vi "TCP_SetControl.vi"(0 "VI Refnum":refnum<vi>, 1 "Input":string, 3 "error in (no error)":errorcluster) -> (8 "Found?":bool, 10 "error out":errorcluster)   [LabVIEW 2019]
uses:
  <vilib>/Utility/Data Type/NI_Data Type.lvlib
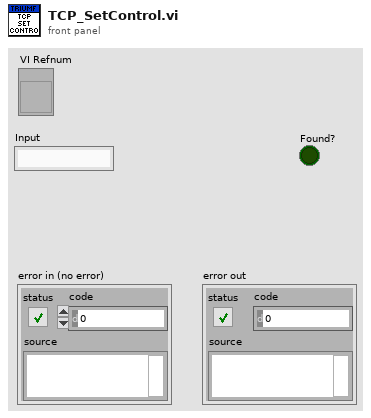
[diagram p1: front panel]
types:
  T1 = typedef "NI_Data Type.lvlib/Data Type.ctl" = enum8{"Invalid Type", "Void", "I8", "I16", "I32", "I64", "U8", "U16", "U32", "U64", "Single Float", "Double Float", "Extended Float", "Single Complex", "Double Complex", "Extended Complex", "Enum U8", "Enum U16", "Enum U32", "Enum U64", "Single Float With Unit", "Double Float With Unit", "Extended Float With Unit", "Single Complex with Unit", "Double Complex with Unit", "Extended Complex with Unit", "Boolean", "String", "Path", "Picture", "Tag", "Array", "Cluster", "Variant", "LV Variant", "Waveform", "Timestamp", "Digital Waveform", "Digital Data", "ExpressData", "Refnum", "External Data", "VI", "Poly VI", "LabVIEW Class Instance", "Fixed Point", "Set Collection", "Map Collection"}
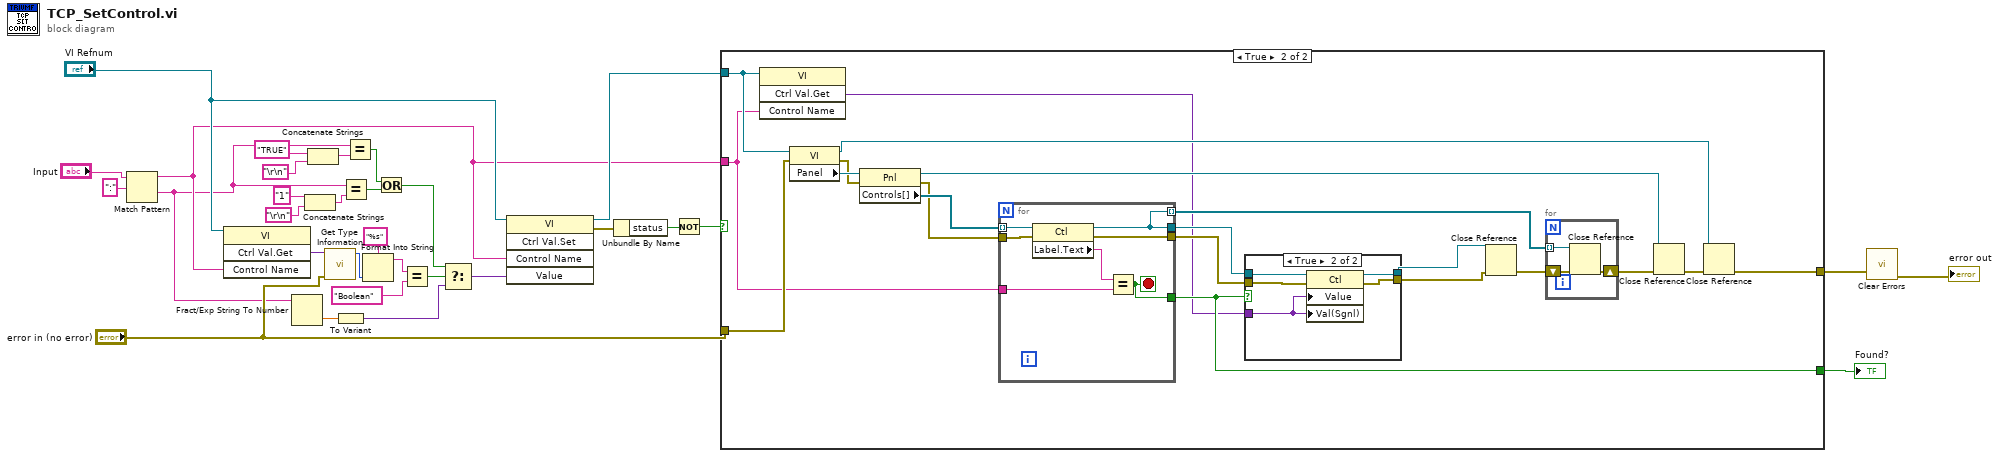
[diagram p0: block diagram]
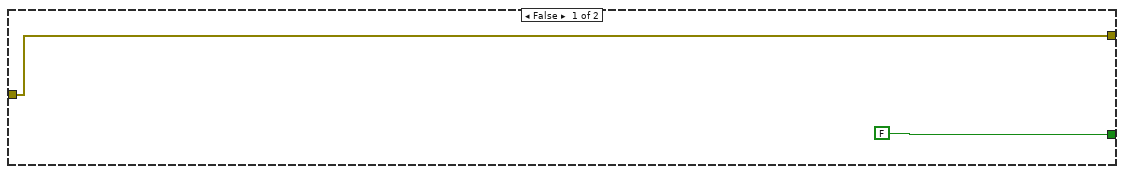
[diagram p2: hidden frame]
diagram:
  n1 = Match Pattern(string="Input", regular expression=":") -> (before substring=w10:string, after substring=w7:string)  [unwired: 1 in, 2 out]
  n2 = invoke class="VI" method="Ctrl Val.Get"(reference="VI Refnum", "Control Name"=w10) -> ("Get Control Value Variant"=w25:variant)  [unwired: 2 in, 3 out]
  n3 = Fract/Exp String To Number(string=w7) -> (number=w17:dbl)  [unwired: 3 in, 1 out]
  n4 = Concatenate Strings("1" ("y"), "\r\n") -> (w1:string)
  n5 = Concatenate Strings("TRUE" ("y"), "\r\n") -> (w4:string)
  n6 = call <vilib>:"Get Type Information.vi"("error in (no error)"="error in (no error)", "variant"=w25) -> ("type"=w8:T1)  [unwired: 5 in, 4 out]
  n7 = To Variant(anything=w17) -> (Variant=w16:variant)
  n8 = Equal?(x=w7, y=w1) -> (x = y?=w22:bool)
  n9 = Equal?(x=w7, y=w4) -> (x = y?=w21:bool)
  n10 = Format Into String(format string="%s", w8) -> (resulting string=w23:string)  [unwired: 2 in, 1 out]
  n11 = Or(x=w21, y=w22) -> (x .or. y?=w19:bool)
  n12 = Equal?(x=w23, y="Boolean") -> (x = y?=w20:bool)
  n13 = Select(t=w19, s=w20, f=w16) -> (s? t:f=w18:variant)
  n14 = invoke class="VI" method="Ctrl Val.Set"(reference="VI Refnum", "Control Name"=w10, "Value"=w18) -> (reference out=w11:refnum<vi>, error out=w15:errorcluster)  [unwired: 2 in, 3 out]
  n15 = Unbundle By Name(w15) -> ("status"=w14:bool)
  n16 = Not(x=w14) -> (.not. x?=w12:bool)
  n17 = case shown="True" w12 {
    tunnel: [FALSE w48] -> w30
    tunnel: w11 -> [_ w37]
    tunnel: [w32 w47] -> w27
    tunnel: "error in (no error)" -> [w32 w36]
    tunnel: w10 -> [_ w35]
    frame False {
    }
    frame True {
      n18 = invoke class="VI" method="Ctrl Val.Get"(reference=w37, "Control Name"=w35) -> ("Get Control Value Variant"=w38:variant)  [unwired: 2 in, 3 out]
      n19 = property class="VI"(reference=w37, error in=w36) -> (reference out=w53:refnum<vi>, error out=w49:errorcluster, "Panel"=w50:refnum<vi>)
      n20 = property class="Pnl"(reference=w50, error in=w49) -> (reference out=w52:refnum<vi>, error out=w40:errorcluster, "Controls[]"=w41:refnum<vi>[])
      n21 = for {
        tunnel: w41 -> [w70] mode=indexing
        tunnel: [w69] -> w45 mode=indexing
        tunnel: [w69] -> w46
        tunnel: [w68] -> w43
        tunnel: w35 -> [w67]
        tunnel: w40 -> [w66]
        tunnel: [w64] -> w48
        stop <- w64 stop-if-true
        n22 = property class="Ctl"(reference=w70, error in=w66) -> (reference out=w69:refnum<vi>, error out=w68:errorcluster, "Label.Text"=w65:string)
        n23 = Equal?(x=w65, y=w67) -> (x = y?=w64:bool)
      }
      n24 = case shown="True" w48 {
        tunnel: [w55 w60] -> w34
        tunnel: w46 -> [w55 w59]
        tunnel: w43 -> [w54 w58]
        tunnel: [w54 w57] -> w42
        tunnel: w38 -> [_ w56]
        frame False {
        }
        frame True {
          n25 = property class="Ctl"(reference=w59, error in=w58, "Value"=w56, "Val(Sgnl)"=w56) -> (reference out=w60:refnum<vi>, error out=w57:errorcluster)
        }
      }
      n26 = Close Reference(reference=w34, error in (no error)=w42) -> (error out=w44:errorcluster)
      n27 = for {
        tunnel: w45 -> [w63] mode=indexing
        shift-right: [w62] -> w39
        shift-left: w44 -> [w61]
        n28 = Close Reference(reference=w63, error in (no error)=w61) -> (error out=w62:errorcluster)
      }
      n29 = Close Reference(reference=w52, error in (no error)=w39) -> (error out=w51:errorcluster)
      n30 = Close Reference(reference=w53, error in (no error)=w51) -> (error out=w47:errorcluster)
    }
  }
  "Found?" <- w30
  n31 = call <vilib>:"Clear Errors.vi"("error in (no error)"=w27) -> ("error out"=→"error out":errorcluster)  [unwired: 5 in, 1 out]
